vi "836_MultiCameraBackground Loop (Brian Turner's conflicted copy 2017-02-17).vi"(10 "port":u16=1180, 11 "CameraDevRef":T1) -> ()   [LabVIEW 2016]
doc: "This VI acquires the image buffer from the camera MJPG stream at the configured fps rate. It notifies any waiting VIs and allows them to pick up the latest image. This allows the camera and robot vision loop to run at different rates. The 1011, camera is far more efficient using MJPGs, and generally, this is probably the better choice for the camera loop.\n \nThis software is licensed. Open the labview\\readme\\WPI Robotics Library Open Source License.txt file for more information."
uses:
  <vilib>/Rock Robotics/WPI/Camera/WPI_CameraSettings Operations.ctl
  <vilib>/Rock Robotics/WPI/Camera/WPI_CameraDevRef.ctl
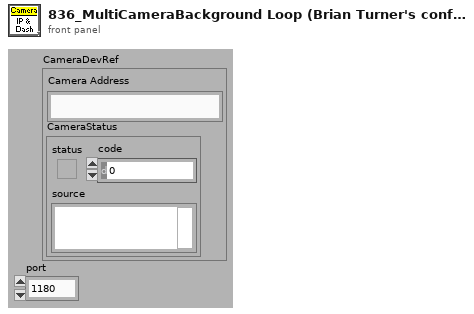
[diagram p1: front panel]
types:
  T1 = typedef "WPI_CameraDevRef.ctl" = cluster{"Camera Address":string, "CameraStatus":errorcluster}
  T2 = typedef "WPI_CameraSettings Operations.ctl" = enum16{"Udate FPS", "Update Compression", "Update Size", "Update White Balance", "Update Brightness", "Update Sharpness", "Update Exposure", "Update Exposure Value", "Update Color Level", "Update Exp Priority", "Update Color Enable", "Update JPG", "Update MJPG", "Read and Clear", "Read", "Init"}
  T3 = typedef "WPI_CameraSettings Control.ctl" = cluster{"FPS":i32, "Compression":i32, "Size":i32, "White Balance":i32, "Brightness":i32, "Sharpness":i32, "Exposure":i32, "Color Level":i32, "Exposure Priority":i32, "Color Enable":i32, "JPG Loop":i32, "MJPG Loop":i32, "Exposure Value":i32}
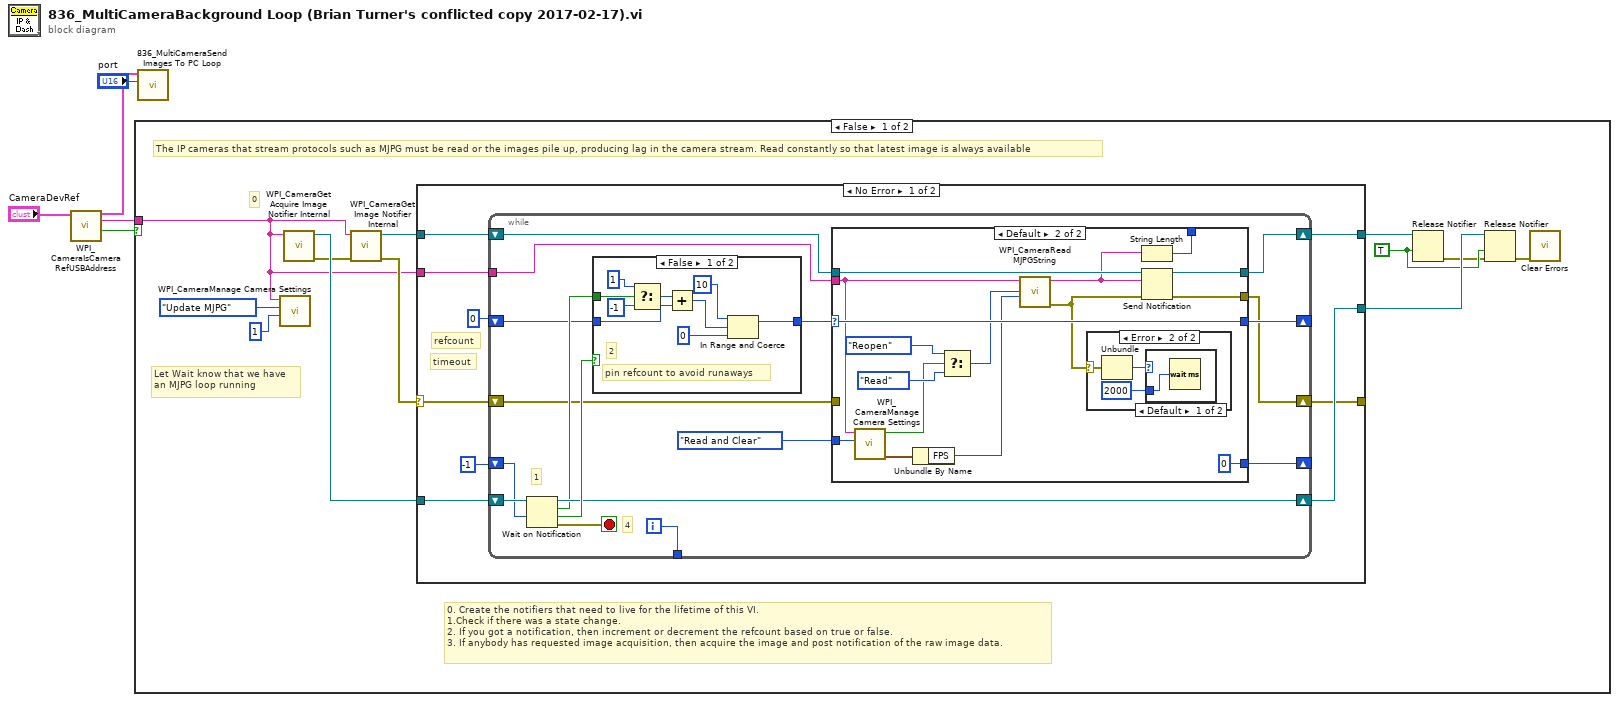
[diagram p0: block diagram]
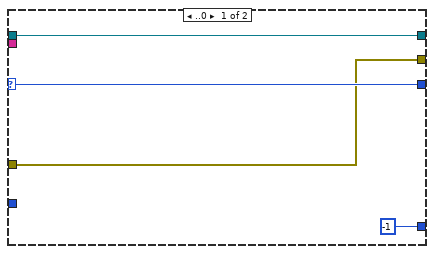
[diagram p2: hidden frame]
diagram:
  n1 = call <vilib>:"WPI_CameraIsCameraRefUSBAddress.vi"("CameraDevRef"="CameraDevRef") -> ("USB?"=w4:bool, "Camera Address Out"=w3:string, "CameraDevRef out"=w2:T1)  [unwired: 7 in, 1 out]
  n2 = case shown="False" w4 {
    tunnel: w3 -> [w7 _]
    frame False {
      w14 = TRUE ("force destroy? (F)")
      # "The IP cameras that stream protocols such as MJPG must be read or the images pile up, producing lag in the camera stream. Read constantly so that latest image is always available"
      # "0. Create the notifiers that need to live for the lifetime of this VI. \n1.Check if there was a state change.\n2. If you got a notification, then increment or decrement the refcount based on true or false.\n3. If anybody has requested image acquisition, then acquire the image and post notification of the raw image data."
      # "Let Wait know that we have\nan MJPG loop running"
      # "0"
      n3 = call <vilib>:"WPI_CameraManage Camera Settings.vi"("Value"=1, "Operation"=WPI_CameraSettings_Operations."Update MJPG", "Camera IP"=w7) -> ()  [unwired: 7 in, 2 out]
      n4 = call <vilib>:"WPI_CameraGet Acquire Image Notifier Internal.vi"("Camera Address"=w7) -> ("error out"=w11:errorcluster, "Acquire Image Notifier"=w12:refnum<notifier>)  [unwired: 1 in, 8 out]
      n5 = call <vilib>:"WPI_CameraGet Image Notifier Internal.vi"("error in (no error)"=w11, "Camera Address"=w7) -> ("error out"=w13:errorcluster, "Image Notifier"=w15:refnum<notifier>)  [unwired: 8 out]
      n6 = case shown="No Error" w13 {
        selector: w13 -> [w19 w80]
        tunnel: w7 -> [w26 _]
        tunnel: w12 -> [w25 w78]
        tunnel: w15 -> [w23 w79]
        tunnel: [w21 w79] -> w17
        tunnel: [w20 w78] -> w16
        tunnel: [w18 w80] -> _
        frame No Error {
          # "timeout"
          # "refcount"
          n7 = while {
            shift-right: [w41] -> w20
            shift-left: w25 -> [w43]
            tunnel: w26 -> [w38]
            shift-right: [w30] -> _
            shift-left: 0 -> [w39]
            shift-right: [w36] -> w21
            shift-left: w23 -> [w37]
            shift-right: [w34] -> _
            shift-left: -1 -> [w35]
            shift-right: [w29] -> w18
            shift-left: w19 -> [w32]
            tunnel: [w27] -> _
            i -> [w27]
            stop <- w33 stop-if-true
            # "4"
            # "1"
            n8 = Wait on Notification(notifier=w43, timeout in ms (-1)=w35) -> (notifier out=w41:refnum<notifier>, notification=w40:bool, timed out?=w42:bool, error out=w33:errorcluster)  [unwired: 1 in, 1 out]
            n9 = case shown="False" w42 {
              tunnel: w40 -> [w76 _]
              tunnel: w39 -> [w72 w77]
              tunnel: [w68 w77] -> w31
              frame False {
                # "pin refcount to avoid runaways"
                # "2"
                n10 = Select(t=1, s=w76, f=-1) -> (s? t:f=w73:i32)
                n11 = Add(x=w73, y=w72) -> (x+y=w69:i32)
                n12 = In Range and Coerce(upper limit=10, x=w69, lower limit=0) -> (coerced(x)=w68:i32)  [unwired: 1 out]
              }
              frame True {
              }
            }
            n13 = case shown="Default" w31 {
              selector: w31 -> [w46 w60]
              tunnel: w38 -> [_ w48]
              tunnel: w37 -> [w47 w63]
              tunnel: [w47 w62] -> w36
              tunnel: [-1 0] -> w34
              tunnel: w32 -> [w44 _]
              tunnel: [w46 w60] -> w30
              tunnel: [w44 w59] -> w29
              tunnel: [_ w53] -> _
              tunnel: WPI_CameraSettings_Operations."Read and Clear" ("Operation") -> [_ w49]
              frame ..0 {
              }
              frame Default {
                n14 = call <vilib>:"WPI_CameraManage Camera Settings.vi"("Operation"=w49, "Camera IP"=w48) -> ("Values"=w51:T3, "Changed"=w52:bool)  [unwired: 8 in]
                n15 = Unbundle By Name(w51) -> ("FPS"=w50:i32)
                n16 = Select(t=enum16{"Read", "Reopen", "Close"}."Reopen" ("Operation"), s=w52, f=enum16{"Read", "Reopen", "Close"}."Read" ("Operation")) -> (s? t:f=w55:enum16{"Read", "Reopen", "Close"})
                n17 = call <vilib>:"WPI_CameraRead MJPGString.vi"("fps"=w50, "Operation"=w55, "address"=w48) -> ("error out"=w58:errorcluster, "Raw Image Data"=w54:string)  [unwired: 7 in]
                n18 = case shown="Error" w58 {
                  selector: w58 -> [_ w66]
                  frame No Error {
                  }
                  frame Error {
                    n19 = Unbundle(w66) -> ("code"=w65:i32)  [unwired: 2 out]
                    n20 = case shown="Default" w65 {
                      tunnel: u32 2000 ("milliseconds to wait") -> [w67 _]
                      frame Default {
                        n21 = Wait (ms)(milliseconds to wait=w67) -> ()  [unwired: 1 out]
                      }
                      frame 56 {
                      }
                    }
                  }
                }
                n22 = String Length(string=w54) -> (length=w53:i32)
                n23 = Send Notification(notification=w54, notifier=w63, error in (no error)=w58) -> (notifier out=w62:refnum<notifier>, error out=w59:errorcluster)
              }
            }
          }
        }
        frame Error {
        }
      }
      n24 = Release Notifier(notifier=w17, force destroy? (F)=w14) -> (error out=w10:errorcluster)  [unwired: 1 in, 2 out]
      n25 = Release Notifier(notifier=w16, force destroy? (F)=w14, error in (no error)=w10) -> (error out=w6:errorcluster)  [unwired: 2 out]
      n26 = call <vilib>:"Clear Errors.vi"("error in (no error)"=w6) -> ()  [unwired: 1 in, 6 out]
    }
    frame True {
      # "The USB cameras may need to be forwarded over ethernet. Read, compress, and send to the Dashbd."
    }
  }
  n27 = call "836_MultiCameraSend Images To PC Loop.vi"("port"="port", "CameraDevRef"=w2) -> ()  [unwired: 10 in]
